vi "Knob Turn.vi"(0 "GEA2 Reference In":refnum<k24>, 7 "Button":T1=enum."Position 1", 11 "Error In":errorcluster) -> (4 "GEA2 Reference Out":refnum<k24>, 15 "Error Out":errorcluster)   [LabVIEW 2018, in "2015 VA Washer.lvlib"]
uses:
  Projects/2015 VA Washer.lvlib
  type defs/Encoder Position.ctl
  D:/Common/LabVIEW GEA2 Toolkit/source/GEA3 DLL Source/GeaCommunication.dll
  Common/LabVIEW GEA2 Toolkit/source/GEA3 DLL Source/GeaCommunication.dll
  Common/LabVIEW GEA2 Toolkit/GEA3/type defs/Source_Destination.ctl
  Common/LabVIEW GEA2 Toolkit/GEA3/type defs/ERD Write Data In.ctl
  Common/LabVIEW GEA2 Toolkit/GEA3/type defs/Data Type.ctl
  C:/Users/iallatyp/Desktop/New folder/GEA3/library/GEA2_Toolkit.lvlib
panel:
  in  "Standalone?":bool
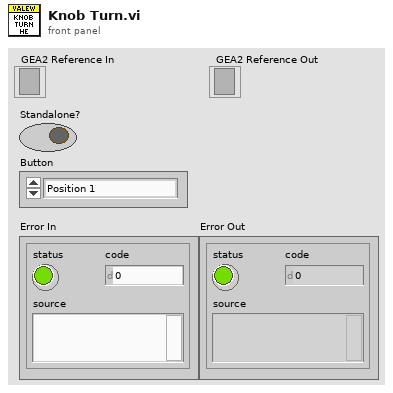
[diagram p1: front panel]
types:
  T1 = typedef "2015 VA Washer.lvlib/Encoder Position.ctl" = enum16{"Position 0", "Position 1", "Position 2", "Position 3", "Position 4", "Position 5", "Position 6", "Position 7", "Position 8", "Position 9", "Position 10", "Position 11", "Position 12", "Position 13", "Clear / Reset"}
  T2 = typedef "GEA2_Toolkit.lvlib/ERD Write Data In.ctl" = cluster{"ERD Number":u16, "Data Type":T3, "Data":string}
  T3 = typedef "GEA2_Toolkit.lvlib/Data Type.ctl" = enum16{"string", "boolean", "uint8_t", "uint16_t", "uint32_t", "uint64_t", "int8_t", "int16_t", "int32_t", "int64_t"}
  T4 = typedef "GEA2_Toolkit.lvlib/Source_Destination.ctl" = cluster{"Source":u8, "Destination":u8}
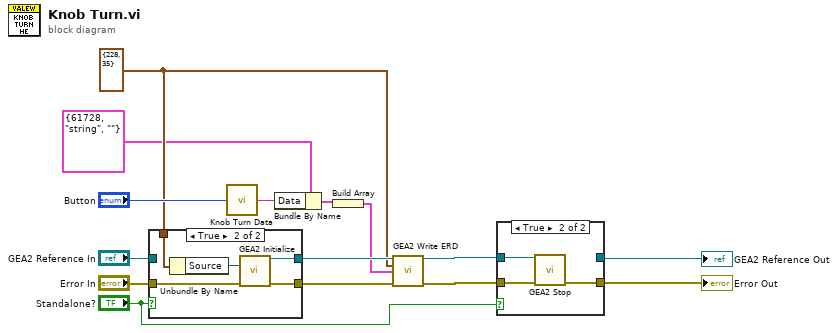
[diagram p0: block diagram]
diagram:
  w3 = T4 {"Source"=228, "Destination"=35} ("GEA Inputs")
  n1 = case shown="True" "Standalone?" {
    tunnel: "Error In" -> [w16 w22]
    tunnel: [w16 w21] -> w9
    tunnel: "GEA2 Reference In" -> [w17 _]
    tunnel: [w17 w20] -> w7
    tunnel: w3 -> [_ w18]
    frame False {
    }
    frame True {
      n2 = Unbundle By Name(w18) -> ("Source"=w19:u8)
      n3 = call "GEA2 Initialize.vi"("Source Address"=w19, "error in"=w22) -> ("GEA2 Reference Out"=w20:refnum<k24>, "error out"=w21:errorcluster)  [unwired: 11 in, 1 out]
    }
  }
  n4 = call "Knob Turn Data.vi"("Switch"="Button") -> ("Switch Message"=w6:string)  [unwired: 14 in]
  n5 = Bundle By Name(cluster=T2 {"ERD Number"=61728, "Data Type"=enum."string", "Data"=""} ("ERD Write Data In"), "Data"=w6) -> (w5:T2)
  n6 = Build Array(w5) -> (w4:T2[])
  n7 = call "GEA2 Write ERD.vi"("GEA2 Reference In"=w7, "GEA Inputs"=w3, "Write ERD List"=w4, "Error In"=w9) -> ("GEA2 Reference Out"=w2:refnum<k24>, "Error Out"=w8:errorcluster)  [unwired: 9 in, 1 out]
  n8 = case shown="True" "Standalone?" {
    tunnel: [w23 w27] -> w12
    tunnel: w2 -> [w24 w26]
    tunnel: [w24 _] -> w11
    tunnel: w8 -> [w23 w25]
    frame False {
    }
    frame True {
      n9 = call "GEA2 Stop.vi"("GEA2 Reference In"=w26, "Error In"=w25) -> ("Error Out"=w27:errorcluster)  [unwired: 13 in]
    }
  }
  "Error Out" <- w12
  "GEA2 Reference Out" <- w11
